vi "Kaelus PIM Validate Stimulus.vi"(9 "Driver Configuration":T1 {"Calibration Date" format="%.2f"; "Parameters"."TX2pmax" format="%.1f"; "Parameters"."TX1pmax" format="%.1f"; "Parameters"."RXstop" format="%.1f"; "Parameters"."RXstart" format="%.1f"; "Parameters"."TX2stop" format="%.1f"; "Parameters"."TX2start" format="%.1f"; "Parameters"."TX1stop" format="%.1f"; "Parameters"."TX1start" format="%.1f"}, 11 "Stimulus":T3 {"Measurement Setup"."TXStep" items=[".2", ".4", "1.0", "2.0"]; "Measurement Parameters"."Direction" items=["Reverse", "Forward", "Auxiliary"]; "Measurement Parameters"."IM Order" items=["3rd", "5th", "7th", "9th", "11th", "13th", "15th", "17th", "19th", "21st", "23rd", "25th", "27th", "29th", "31st", "33rd"]; "Measurement Parameters"."Averaging" items=["None", "Minimum", "Normal", "High", "Maximum"]}) -> (3 "Validate Variant":string)   [LabVIEW 2011]
uses:
  PIM Stimulus.ctl
  PIM Cmd Params.ctl
  BPIMCore/HW IO/IMOrder.ctl
  BPIMCore/HW IO/HW Averaging.ctl
  BPIMCore/HW IO/MeasMode.ctl
  BPIMCore/Display/display_unit_format.ctl
  BPIMCore/HW IO/DUTport.ctl
  BPIMCore/HW IO/PIM Sweep Step Size.ctl
  PIM Configuration.ctl
  PIM Interface Language.ctl
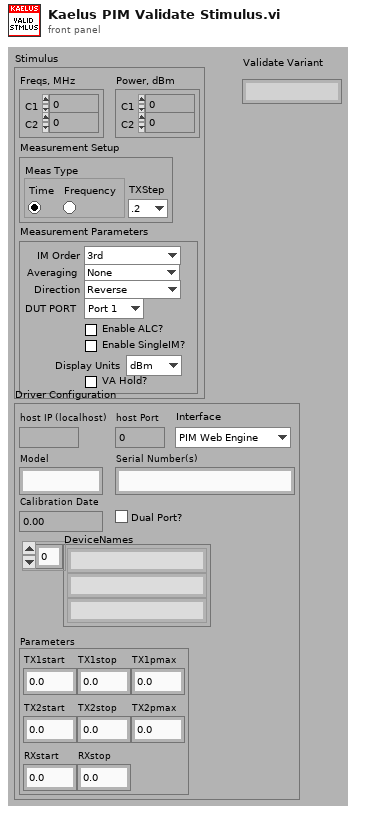
[diagram p1: front panel]
types:
  T1 = typedef "PIM Configuration.ctl" = cluster{"host IP (localhost)":string, "host Port":u16, "Model":string, "Serial Number(s)":string, "Calibration Date":dbl, "Dual Port?":bool, "DeviceNames":string[], "Parameters":cluster{"TX1start":dbl, "TX1stop":dbl, "TX1pmax":dbl, "TX2start":dbl, "TX2stop":dbl, "TX2pmax":dbl, "RXstart":dbl, "RXstop":dbl}, "Interface":T2}
  T2 = typedef "PIM Interface Language.ctl" = enum16{"PIM Web Engine", "PIM HW Engine"}
  T3 = typedef "PIM Stimulus.ctl" = cluster{"Carrier Frequencies":cluster{"C1 Freq, MHz":dbl, "C2 Freq, MHz":dbl}, "Carrier Powers":cluster{"C1 Power,dBm":dbl, "C2 Power, dBm":dbl}, "Measurement Parameters":T4, "Measurement Setup":cluster{"Meas Type":enum32{"Time", "Frequency"}, "TXStep":T10}}
  T4 = typedef "PIM Cmd Params.ctl" = cluster{"IM Order":T5, "Averaging":T6, "Direction":T7, "Enable ALC?":bool, "Enable SingleIM?":bool, "Display Units":T8, "VA Hold?":bool, "DUT PORT":T9}
  T5 = typedef "IMOrder.ctl" = u8
  T6 = typedef "HW Averaging.ctl" = u16
  T7 = typedef "MeasMode.ctl" = u16
  T8 = typedef "display_unit_format.ctl" = enum16{"dBm", "dBc"}
  T9 = typedef "DUTport.ctl" = enum16{"Port 1", "Port 2"}
  T10 = typedef "PIM Sweep Step Size.ctl" = u16
  T11 = enum16{"Carrier 1 Frequency", "Carrier 2 Frequency", "Carrier 1 Power", "Carrier 2 Power", "Measurement Port"}[]
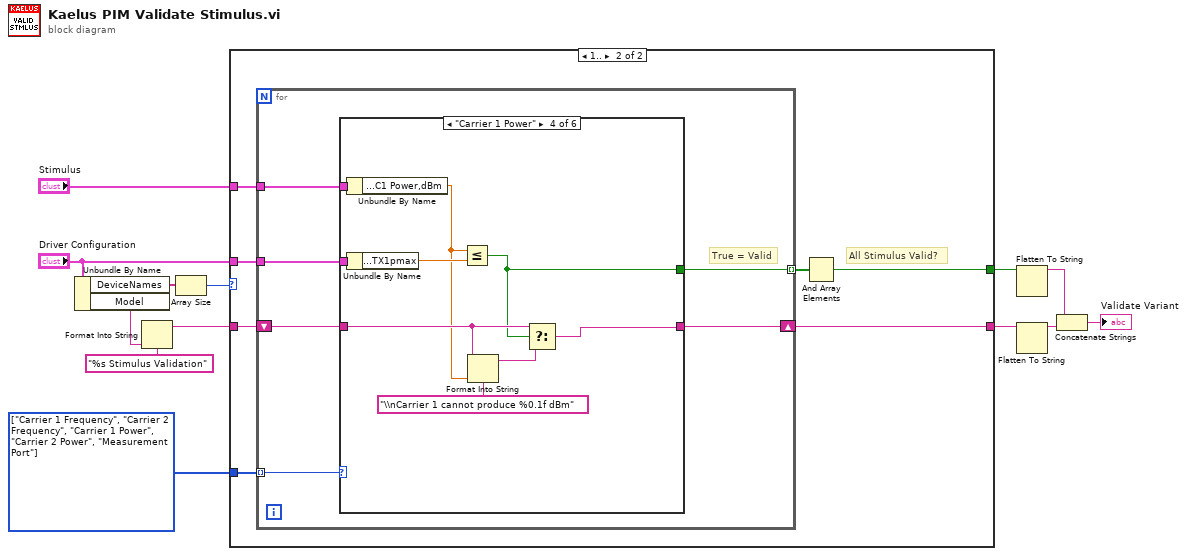
[diagram p0: block diagram]
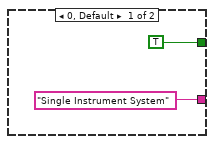
[diagram p2: hidden frame]
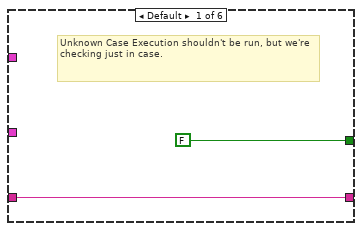
[diagram p3: hidden frame]
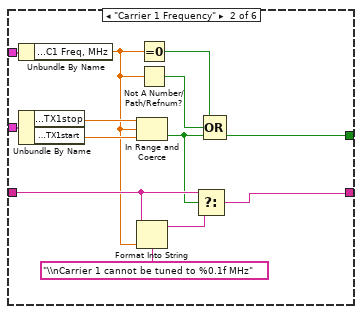
[diagram p4: hidden frame]
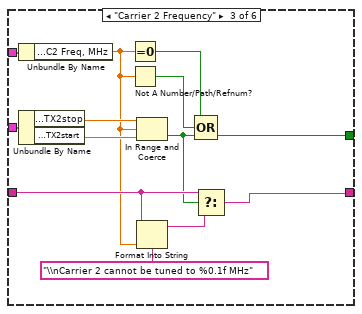
[diagram p5: hidden frame]
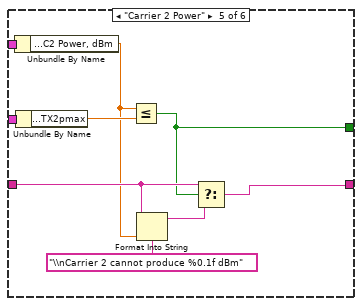
[diagram p6: hidden frame]
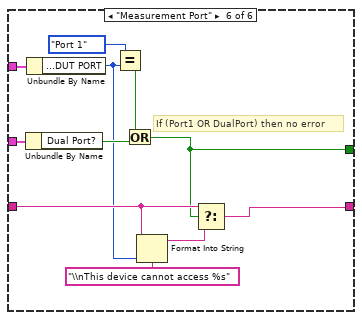
[diagram p7: hidden frame]
diagram:
  w10 = T11 [enum."Carrier 1 Frequency", enum."Carrier 2 Frequency", enum."Carrier 1 Power", enum."Carrier 2 Power", enum."Measurement Port"] items=["Carrier 1 Frequency", "Carrier 2 Frequency", "Carrier 1 Power", "Carrier 2 Power", "Measurement Port"]
  n1 = Unbundle By Name("Driver Configuration") -> ("DeviceNames"=w2:string[], "Model"=w6:string)
  n2 = Format Into String(format string="%s Stimulus Validation", w6) -> (resulting string=w5:string)  [unwired: 2 in, 1 out]
  n3 = Array Size(array=w2) -> (size(s)=w1:i32)
  n4 = case shown="1.." w1 {
    tunnel: w10 -> [_ w22]
    tunnel: "Stimulus" -> [_ w21]
    tunnel: "Driver Configuration" -> [_ w20]
    tunnel: w5 -> [_ w19]
    tunnel: ["Single Instrument System" w18] -> w4
    tunnel: [TRUE w16] -> w3
    frame 0, Default {
    }
    frame 1.. {
      # "All Stimulus Valid?"
      n5 = for {
        tunnel: w22 -> [w28] mode=indexing
        tunnel: w21 -> [w27]
        tunnel: w20 -> [w26]
        shift-right: [w24] -> w18
        shift-left: w19 -> [w25]
        tunnel: [w23] -> w17 mode=indexing
        # "True = Valid"
        n6 = case shown="\"Carrier 1 Power\"" w28 {
          tunnel: w27 -> [_ w43 w56 w65 w74 w85]
          tunnel: w26 -> [_ w42 w55 w64 w73 w84]
          tunnel: w25 -> [w30 w38 w51 w62 w71 w83]
          tunnel: [w30 w36 w49 w60 w69 w81] -> w24
          tunnel: [FALSE w31 w44 w57 w66 w75] -> w23
          frame Default {
            # "Unknown Case Execution shouldn't be run, but we're checking just in case."
          }
          frame "Carrier 1 Frequency" {
            n7 = Unbundle By Name(w43) -> ("Carrier Frequencies.C1 Freq, MHz"=w35:dbl)
            n8 = Unbundle By Name(w42) -> ("Parameters.TX1stop"=w40:dbl, "Parameters.TX1start"=w39:dbl)
            n9 = In Range and Coerce(upper limit=w40, x=w35, lower limit=w39) -> (In Range?=w34:bool)  [unwired: 1 out]
            n10 = Format Into String(format string="\\nCarrier 1 cannot be tuned to %0.1f MHz", initial string=w38, w35) -> (resulting string=w37:string)  [unwired: 1 in, 1 out]
            n11 = Equal To 0?(x=w35) -> (x = 0?=w32:bool)
            n12 = Not A Number/Path/Refnum?(number/path/refnum=w35) -> (NaN/Path/Refnum?=w33:bool)
            n13 = Select(t=w38, s=w34, f=w37) -> (s? t:f=w36:string)
            n14 = Compound Arithmetic op=OR(w32, w33, w34) -> (w31:bool)
          }
          frame "Carrier 2 Frequency" {
            n15 = Unbundle By Name(w56) -> ("Carrier Frequencies.C2 Freq, MHz"=w48:dbl)
            n16 = Unbundle By Name(w55) -> ("Parameters.TX2stop"=w53:dbl, "Parameters.TX2start"=w52:dbl)
            n17 = Equal To 0?(x=w48) -> (x = 0?=w46:bool)
            n18 = Not A Number/Path/Refnum?(number/path/refnum=w48) -> (NaN/Path/Refnum?=w47:bool)
            n19 = In Range and Coerce(upper limit=w53, x=w48, lower limit=w52) -> (In Range?=w45:bool)  [unwired: 1 out]
            n20 = Format Into String(format string="\\nCarrier 2 cannot be tuned to %0.1f MHz", initial string=w51, w48) -> (resulting string=w50:string)  [unwired: 1 in, 1 out]
            n21 = Compound Arithmetic op=OR(w46, w47, w45) -> (w44:bool)
            n22 = Select(t=w51, s=w45, f=w50) -> (s? t:f=w49:string)
          }
          frame "Carrier 1 Power" {
            n23 = Unbundle By Name(w65) -> ("Carrier Powers.C1 Power,dBm"=w58:dbl)
            n24 = Unbundle By Name(w64) -> ("Parameters.TX1pmax"=w59:dbl)
            n25 = Less Or Equal?(x=w58, y=w59) -> (x <= y?=w57:bool)
            n26 = Format Into String(format string="\\nCarrier 1 cannot produce %0.1f dBm", initial string=w62, w58) -> (resulting string=w61:string)  [unwired: 1 in, 1 out]
            n27 = Select(t=w62, s=w57, f=w61) -> (s? t:f=w60:string)
          }
          frame "Carrier 2 Power" {
            n28 = Unbundle By Name(w74) -> ("Carrier Powers.C2 Power, dBm"=w67:dbl)
            n29 = Unbundle By Name(w73) -> ("Parameters.TX2pmax"=w68:dbl)
            n30 = Less Or Equal?(x=w67, y=w68) -> (x <= y?=w66:bool)
            n31 = Format Into String(format string="\\nCarrier 2 cannot produce %0.1f dBm", initial string=w71, w67) -> (resulting string=w70:string)  [unwired: 1 in, 1 out]
            n32 = Select(t=w71, s=w66, f=w70) -> (s? t:f=w69:string)
          }
          frame "Measurement Port" {
            # "If (Port1 OR DualPort) then no error"
            n33 = Unbundle By Name(w84) -> ("Dual Port?"=w79:bool)
            n34 = Unbundle By Name(w85) -> ("Measurement Parameters.DUT PORT"=w77:T9)
            n35 = Equal?(x=DUTport."Port 1" ("Measurement Parameters.DUT PORT"), y=w77) -> (x = y?=w80:bool)
            n36 = Or(x=w80, y=w79) -> (x .or. y?=w75:bool)
            n37 = Format Into String(format string="\\nThis device cannot access %s", initial string=w83, w77) -> (resulting string=w82:string)  [unwired: 1 in, 1 out]
            n38 = Select(t=w83, s=w75, f=w82) -> (s? t:f=w81:string)
          }
        }
      }
      n39 = And Array Elements(Boolean array=w17) -> (logical AND=w16:bool)
    }
  }
  n40 = Flatten To String(anything=w3) -> (data string=w12:string)  [unwired: 1 in, 4 out]
  n41 = Flatten To String(anything=w4) -> (data string=w13:string)  [unwired: 1 in, 4 out]
  n42 = Concatenate Strings(w12, w13) -> (→"Validate Variant":string)
